vi "Write Events.vi"(8 "error in (no error)":errorcluster, 10 "Events":T1, 11 "Engine in":refnum<class "Engine.lvclass">) -> (0 "error out":errorcluster, 3 "Engine out":refnum<class "Engine.lvclass">)   [LabVIEW 2019, in "Engine.lvlib" / "Engine.lvclass"]
uses:
  Project/Engine.lvclass
  Custom Controls/Engine Events.ctl
  Custom Controls/System Events.ctl
  Custom Controls/System Status.ctl
  Custom Controls/Manual Events.ctl
  Custom Controls/UUT_Events.ctl
  Custom Controls/Interface Events.ctl
  Project/Engine.lvclass/Engine.ctl
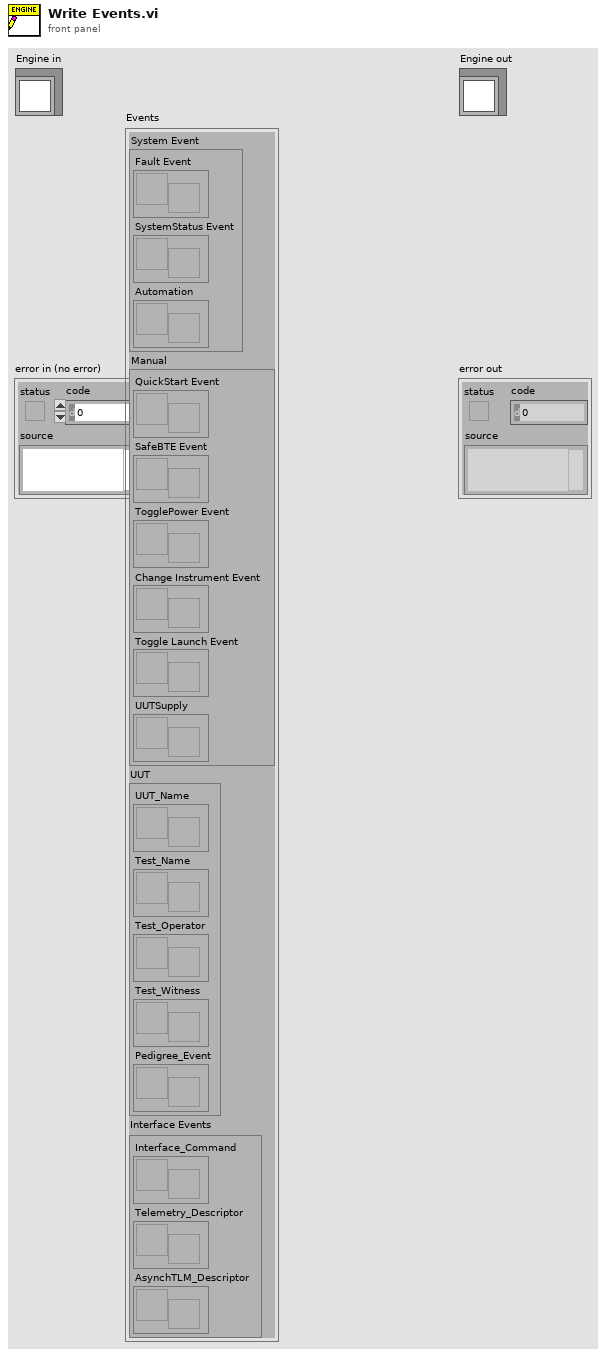
[diagram p1: front panel]
types:
  T1 = typedef "Engine.lvlib/Engine.lvclass/Engine Events.ctl" = cluster{"System Event":T2, "Manual":T3, "UUT":T4, "Interface Events":T5}
  T2 = typedef "Engine.lvlib/Engine.lvclass/System Events.ctl" = cluster{"Fault Event":refnum<user-event>, "SystemStatus Event":refnum<user-event>, "Automation":refnum<user-event>}
  T3 = typedef "Engine.lvlib/Engine.lvclass/Manual Events.ctl" = cluster{"QuickStart Event":refnum<user-event>, "SafeBTE Event":refnum<user-event>, "TogglePower Event":refnum<user-event>, "Change Instrument Event":refnum<user-event>, "Toggle Launch Event":refnum<user-event>, "UUTSupply":refnum<user-event>}
  T4 = typedef "Engine.lvlib/Engine.lvclass/UUT_Events.ctl" = cluster{"UUT_Name":refnum<user-event>, "Test_Name":refnum<user-event>, "Test_Operator":refnum<user-event>, "Test_Witness":refnum<user-event>, "Pedigree_Event":refnum<user-event>}
  T5 = typedef "Engine.lvlib/Engine.lvclass/Interface Events.ctl" = cluster{"Interface_Command":refnum<user-event>, "Telemetry_Descriptor":refnum<user-event>, "AsynchTLM_Descriptor":refnum<user-event>}
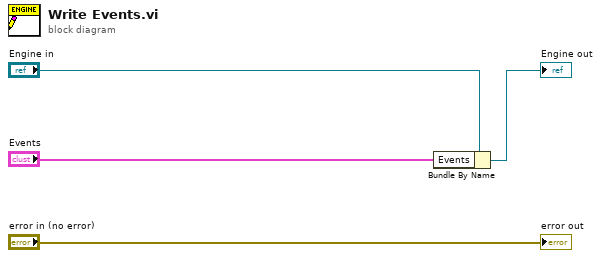
[diagram p0: block diagram]
diagram:
  n1 = Bundle By Name(cluster="Engine in", "Events"="Events") -> (→"Engine out":refnum<class "Engine.lvclass">)
  "error out" <- "error in (no error)"
